vi "LDO_Setup_Parameters.vi"(4 "Temp (°F) - Automatic Mode":dbl=32.0 min=32.0 max=203.0, 5 "Alicat_GasMeter":refnum<queue>, 6 "Valve % Open - Automatic Mode":dbl=15.0 min=15.0 max=100.0, 7 "Modbus":refnum<queue>, 8 "error in (no error)":errorcluster, 11 "UI in":refnum<queue>) -> (0 "error out":errorcluster)   [LabVIEW 2020]
uses:
  Message Queue/Message Cluster.ctl
  Message Queue/Enqueue Message (Single).vi
  Message Queue/Message Queue.lvlib
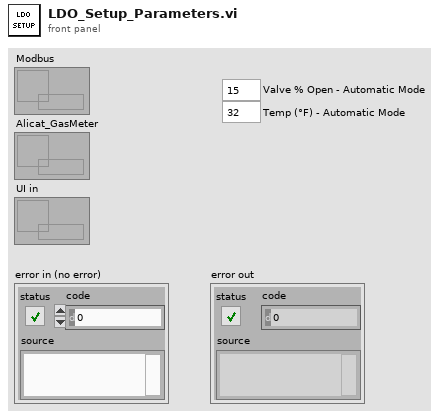
[diagram p1: front panel]
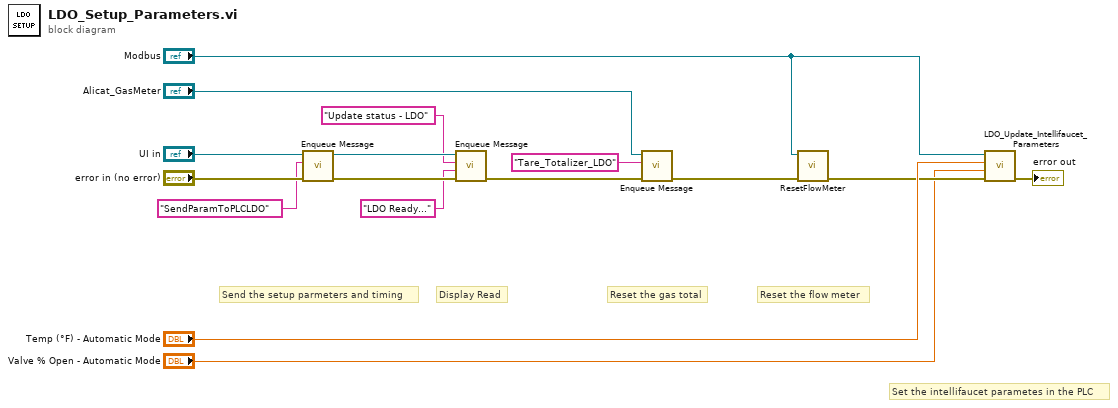
[diagram p0: block diagram]
diagram:
  # "Set the intellifaucet parametes in the PLC"
  # "Reset the flow meter"
  # "Reset the gas total"
  # "Display Read"
  # "Send the setup parmeters and timing"
  n1 = call-poly "Enqueue Message.vi"("error in (no error)"="error in (no error)", "Message"="SendParamToPLCLDO", "Message Queue"="UI in") -> ("error out"=w16:errorcluster, "dup Message Queue"=w14:refnum<queue>)  [unwired: 7 in]
  n2 = call-poly "Enqueue Message.vi"("error in (no error)"=w16, "Message Data"="LDO Ready..." ("Ready..."), "Message"="Update status - LDO", "Message Queue"=w14) -> ("error out"=w7:errorcluster)  [unwired: 6 in, 1 out]
  n3 = call-poly "Enqueue Message.vi"("error in (no error)"=w7, "Message"="Tare_Totalizer_LDO", "Message Queue"="Alicat_GasMeter") -> ("error out"=w6:errorcluster)  [unwired: 7 in, 1 out]
  n4 = call "ResetFlowMeter.vi"("error in (no error)"=w6, "Queue in"="Modbus") -> ("error out 2"=w4:errorcluster)  [unwired: 9 in]
  n5 = call "LDO_Update_Intellifaucet_Parameters.vi"("error in (no error)"=w4, "Valve % Open - Automatic Mode"="Valve % Open - Automatic Mode", "Temp (°F) - Automatic Mode"="Temp (°F) - Automatic Mode", "Modbus Input"="Modbus") -> ("error out"=→"error out":errorcluster)  [unwired: 7 in]
